vi "Create config database.vi"() -> ()   [LabVIEW 2020, in "Sandbox.lvlib"]
uses:
  Sandbox.lvlib
  externals/sqlite3/Source/sqlite3.lvclass/sqlite3.ctl
  externals/sqlite3/Source/sqlite3.lvclass
  D:/Project/Labview-Projects/database-configuration/externals/database-interface/IDatabase/IDatabase/IDatabase.lvclass
  Source/sqlite-queries/sqlite-queries.lvclass
  D:/Project/Labview-Projects/database-configuration/Source/IConfigDBQueries/IConfigurationDatabaseQueries.lvclass
  Source/configuration-database.lvclass
  C:/Program Files/National Instruments/LabVIEW 2020/vi.lib/gpm_packages/@cs/Configuration/Source/IConfiguration/IConfiguration.lvclass
  <vilib>/Utility/error.llb/Error Cluster From Error Code.vi
  <vilib>/gpm_packages/@cs/Configuration/Source/ConfigurationReference/ConfigurationReference.lvclass
panel:
  out "Database metadata":string[][](array[string])
  out "PRAGMA table info":string[][](array[string])
  out "Tables out":string[](array[string])
  in  "Path":path=path "E:/labview/database-interface/sqlite3/test database/new config999.db"
  out "Great success?":bool
  out "error out":errorcluster
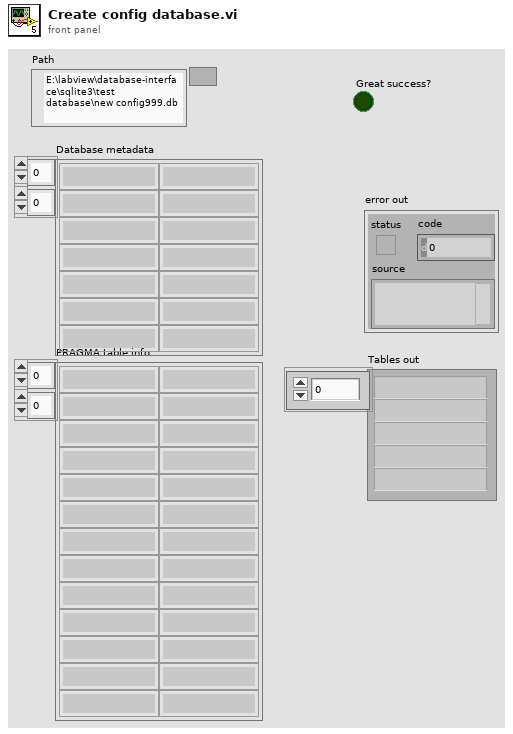
[diagram p1: front panel]
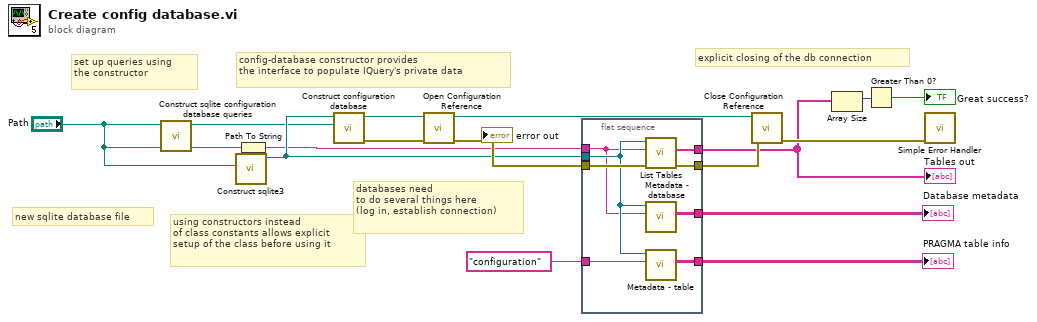
[diagram p0: block diagram]
diagram:
  # "set up queries using \nthe constructor"
  # "new sqlite database file"
  # "explicit closing of the db connection"
  # "databases need\nto do several things here\n(log in, establish connection)"
  # "config-database constructor provides\nthe interface to populate IQuery's private data"
  # "using constructors instead\nof class constants allows explicit\nsetup of the class before using it"
  n1 = call "Construct sqlite configuration database queries.vi"("database path"="Path") -> ("sqlite-configdb-queries out"=w1:refnum<class "sqlite-queries.lvclass">)  [unwired: 9 in, 1 out]
  n2 = call "Construct sqlite3.vi"("DatabaseFilePath"="Path") -> ("sqlite3 out"=w7:refnum<class "sqlite3.lvclass">)  [unwired: 9 in, 1 out]
  n3 = Path To String(path="Path") -> (string=w5:string)
  n4 = call "Construct configuration database.vi"("SQL logic type"=w1, "Database type in"=w7) -> ("error out"=w13:errorcluster, "database-configuration out"=w14:refnum<class "configuration-database.lvclass">)  [unwired: 8 in]
  n5 = call <vilib>:"Open Configuration Reference.vi"("error in (no error)"=w13, "Configuration Type"=w14) -> ("error out"=w11:errorcluster, "Configuration Reference"=w15:refnum<data-value>)  [unwired: 8 in]
  "error out" <- w11
  n6 = flat-sequence {
    tunnel: [w24] -> w12
    tunnel: w11 -> [w23]
    tunnel: [w22] -> w10
    tunnel: w7 -> [w21]
    tunnel: "configuration" ("Table in") -> [w20]
    tunnel: w5 -> [w19]
    tunnel: [w18] -> w3
    tunnel: [w17] -> w4
    frame #0 {
      n7 = call-dynamic "List Tables.vi"("error in (no error)"=w23, "Database in"=w19, "sqlite in"=w21) -> ("error out"=w24:errorcluster, "Tables out"=w22:string[])  [unwired: 6 in, 1 out]
      n8 = call-dynamic "Metadata - database.vi"("Database in"=w19, "IDatabase in"=w21) -> ("Database metadata"=w18:string[][])  [unwired: 7 in, 2 out]
      n9 = call-dynamic "Metadata - table.vi"("Table in"=w20, "sqlite in"=w21) -> ("PRAGMA table info"=w17:string[][])  [unwired: 7 in, 2 out]
    }
  }
  n10 = call <vilib>:"Close Configuration Reference.vi"("error in (no error)"=w12, "Configuration Reference"=w15) -> ("error out"=w16:errorcluster)  [unwired: 9 in]
  n11 = Array Size(array=w10) -> (size(s)=w9:i32)
  n12 = Greater Than 0?(x=w9) -> (x > 0?=→"Great success?":bool)
  n13 = call <vilib>:"Simple Error Handler.vi"("error in (no error)"=w16) -> ()  [unwired: 4 in, 5 out]
  "Tables out" <- w10
  "PRAGMA table info" <- w4
  "Database metadata" <- w3
